vi "DataAndSave.vi"(7 "Proviene de?":enum16{""}(ring), 8 "error in (no error)":errorcluster, 9 "Dato":string, 10 "Path":path, 11 "Guardar TextoPlano in":refnum<class "Guardar TextoPlano.lvclass">) -> (0 "error out":errorcluster, 3 "Guardar TextoPlano out":refnum<class "Guardar TextoPlano.lvclass">)   [LabVIEW 2020, in "Guardar TextoPlano.lvlib" / "Guardar TextoPlano.lvclass"]
uses:
  Guardar TextoPlano.lvclass
  Guardar TextoPlano.lvclass/Guardar TextoPlano.ctl
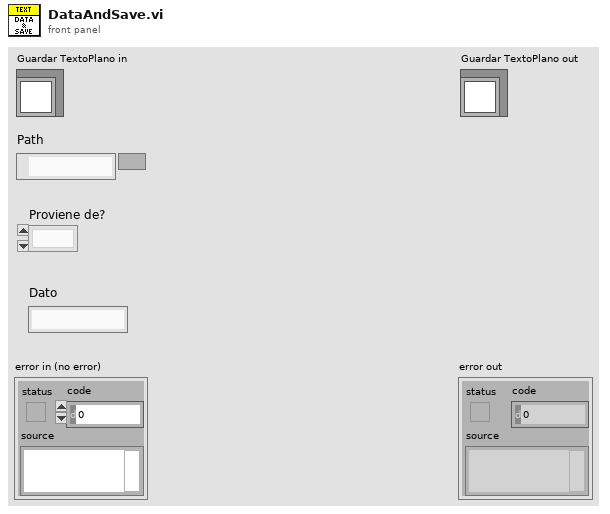
[diagram p1: front panel]
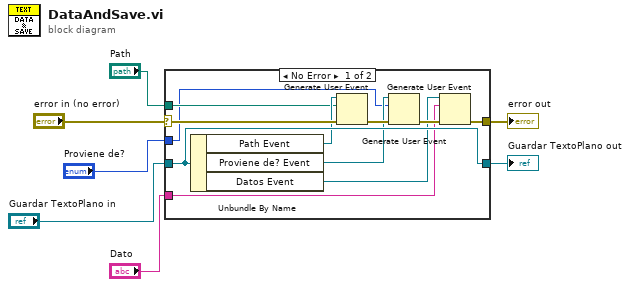
[diagram p0: block diagram]
diagram:
  n1 = case shown="No Error" "error in (no error)" {
    selector: "error in (no error)" -> [w14 w20]
    tunnel: [w15 w20] -> w6
    tunnel: [w18 w19] -> w4
    tunnel: "Guardar TextoPlano in" -> [w18 w19]
    tunnel: "Path" -> [w12 _]
    tunnel: "Proviene de?" -> [w10 _]
    tunnel: "Dato" -> [w9 _]
    frame No Error {
      n2 = Unbundle By Name(w18) -> ("Path Event"=w13:refnum<user-event>, "Proviene de? Event"=w11:refnum<user-event>, "Datos Event"=w8:refnum<user-event>)
      n3 = Generate User Event(user event=w13, event data cluster=w12, error in=w14) -> (error out=w17:errorcluster)  [unwired: 1 in, 1 out]
      n4 = Generate User Event(user event=w11, event data cluster=w10, error in=w17) -> (error out=w16:errorcluster)  [unwired: 1 in, 1 out]
      n5 = Generate User Event(user event=w8, event data cluster=w9, error in=w16) -> (error out=w15:errorcluster)  [unwired: 1 in, 1 out]
    }
    frame Error {
    }
  }
  "error out" <- w6
  "Guardar TextoPlano out" <- w4
